vi "TCP.IP Client for Ripple Detection - Copy.vi"() -> ()   [LabVIEW 2021]
doc: "Demonstrates how to open a connection to an TCP server, read the data being sent, and display the data on a chart. This VI is designed to stop if the TCP connection is terminated."
panel:
  out "Filtered":dbl[](graph)
  out "Array Size 3":u32
  out "Delayed RMS2>RMS1 for 3 data":dynamicdata(graph)
  out "RMS2>RMS1 for 3 data":dynamicdata(graph)
  out "Array Size":u32
  out "RMS2>RMS1":dynamicdata(graph)
  out "RMS1":dynamicdata(graph)
  out "RMS2":dynamicdata(graph)
  out "Raw Data Collected":dynamicdata(graph)
  in  "Boolean":bool
  in  "Server Closed":string="The server VI closed the connection."
  out "Raw Data":dbl[](graph)
  in  "Stop":bool
  # "Overview: Demonstrates the use of the TCP functions to connect to a TCP server VI and receive data.\nInstructions:\n1. Ensure Simple TCP - Server.vi is already running.\n2. Run the VI.\n3. Click Stop to stop the VI. Note that if you stop the server VI, this VI will stop automatically."
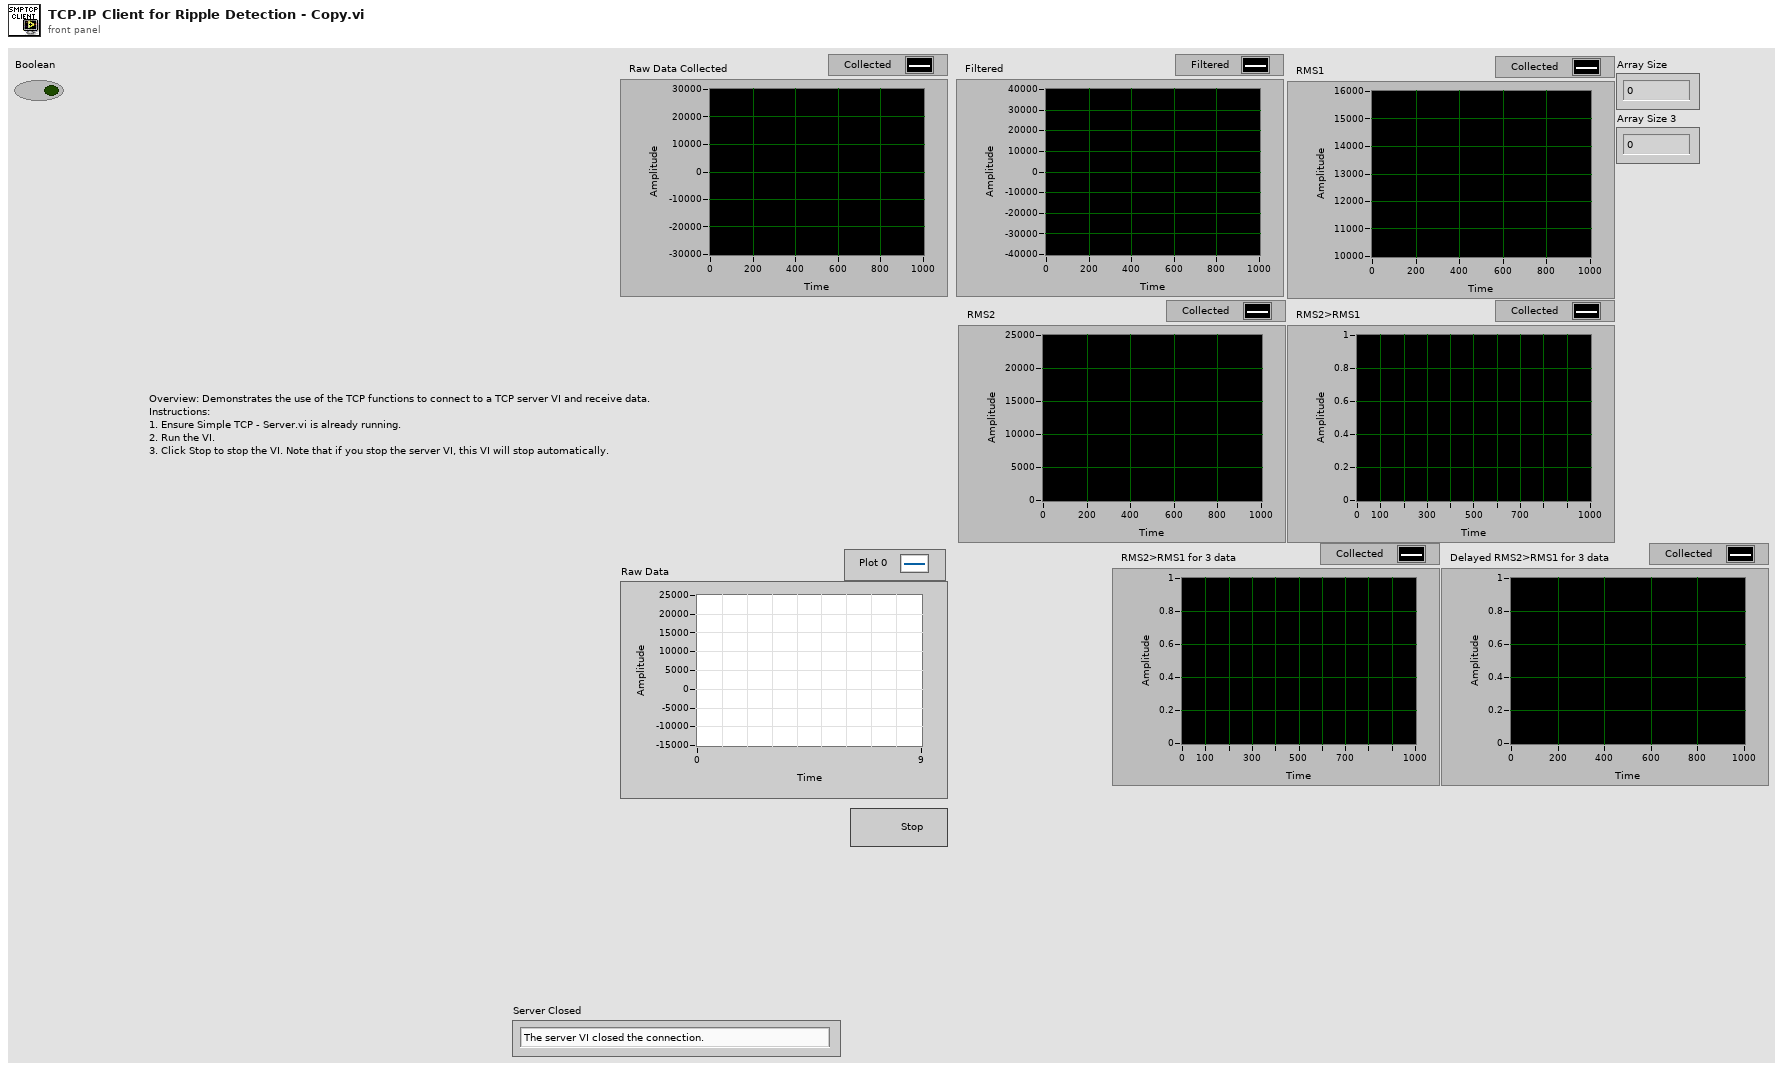
[diagram p1: front panel]
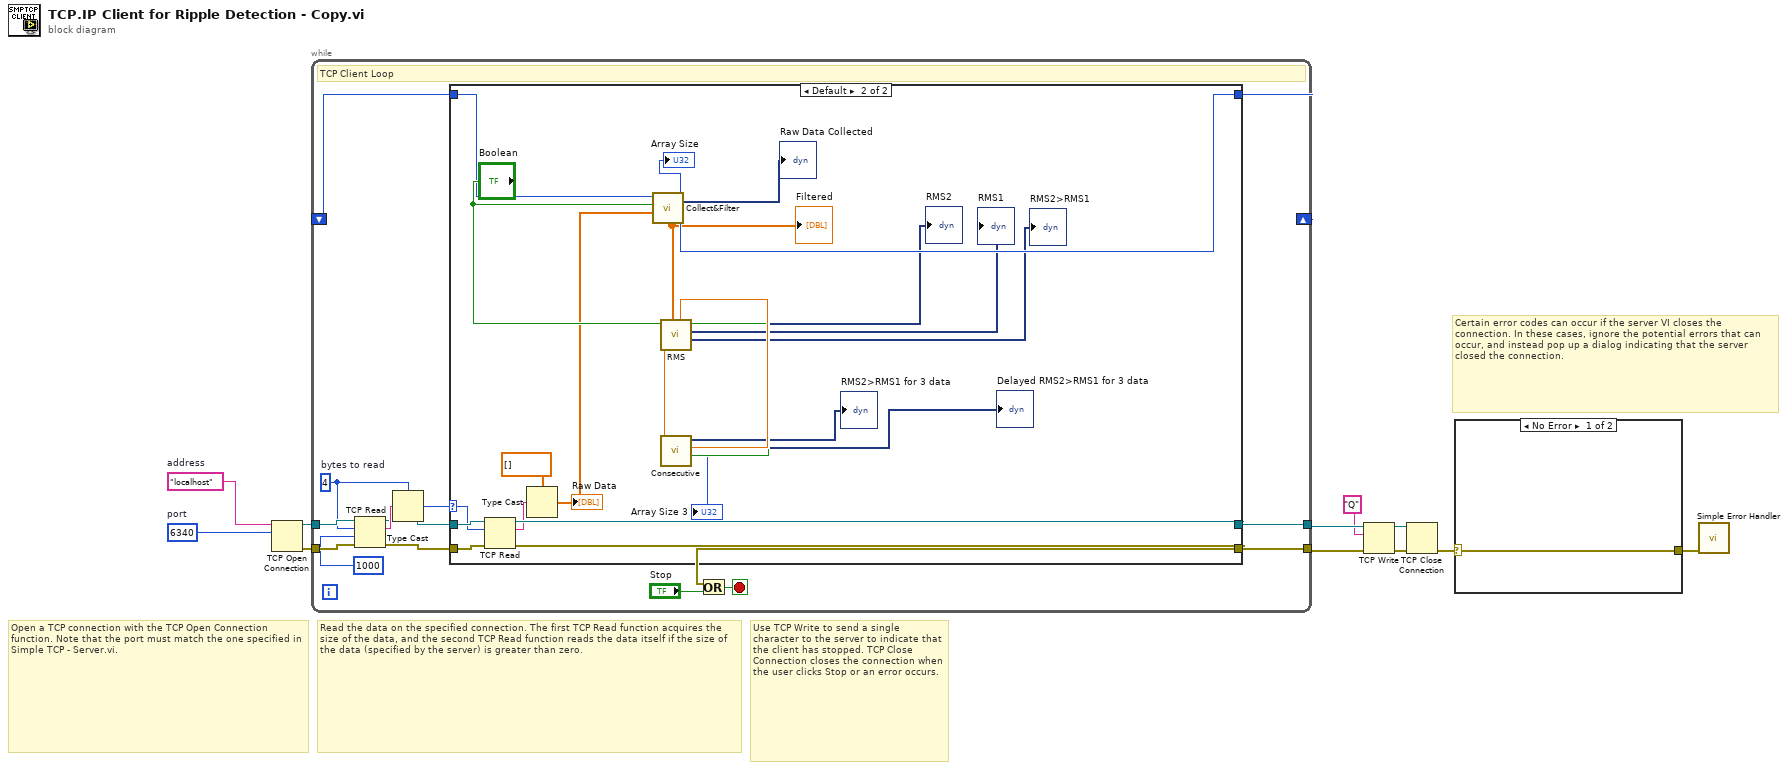
[diagram p0: block diagram]
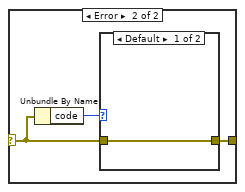
[diagram p2: hidden frame]
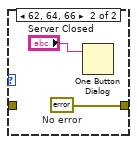
[diagram p3: hidden frame]
diagram:
  w1 = u16 6340  # port
  w2 = "localhost"  # address
  # "Certain error codes can occur if the server VI closes the connection. In these cases, ignore the potential errors that can occur, and instead pop up a dialog indicating that the server closed the connection."
  # "Use TCP Write to send a single character to the server to indicate that the client has stopped. TCP Close Connection closes the connection when the user clicks Stop or an error occurs."
  # "Read the data on the specified connection. The first TCP Read function acquires the size of the data, and the second TCP Read function reads the data itself if the size of the data (specified by the server) is greater than zero."
  # "Open a TCP connection with the TCP Open Connection function. Note that the port must match the one specified in Simple TCP - Server.vi."
  n1 = TCP Open Connection(address=w2, remote port or service name=w1) -> (connection ID=w11:refnum<k5>, error out=w10:errorcluster)  [unwired: 3 in]
  n2 = while {
    tunnel: w10 -> [w21]
    tunnel: w11 -> [w22]
    tunnel: [w17] -> w8
    tunnel: [w16] -> w6
    shift-right: [w12] -> _
    shift-left: _ -> [w13]
    stop <- w18 stop-if-true
    w20 = 4  # bytes to read
    # "TCP Client Loop"
    n3 = TCP Read(connection ID=w22, bytes to read=w20, error in (no error)=w21, 9:1000 ("timeout ms (25000)")) -> (connection ID out=w24:refnum<k5>, data out=w25:string, error out=w23:errorcluster)  [unwired: 1 in]
    n4 = Type Cast(type=w20, x=w25) -> (*(type *) &x=w15:i32)
    n5 = case shown="Default" w15 {
      selector: w15 -> [_ w44]
      tunnel: w24 -> [w28 w50]
      tunnel: w23 -> [w27 w49]
      tunnel: [w28 w47] -> w17
      tunnel: [w27 w46] -> w16
      tunnel: w13 -> [w26 w39]
      tunnel: [w26 w38] -> w12
      frame ..0 {
        # "The server has not written any data"
      }
      frame Default {
        n6 = TCP Read(connection ID=w50, bytes to read=w44, error in (no error)=w49) -> (connection ID out=w47:refnum<k5>, data out=w45:string, error out=w46:errorcluster)  [unwired: 2 in]
        n7 = Type Cast(type=dbl[] [] ("chart"), x=w45) -> (*(type *) &x=w37:dbl[])
        "Raw Data" <- w37
        n8 = call "Collect&Filter.vi"("chart"=w37, "Boolean"="Boolean", "Numeric in"=w39) -> ("Collected Signals"=→"Raw Data Collected":dynamicdata, "Numeric out"=w38:i32, "Array Size"=→"Array Size":u32, "Filtered X"=w29:dbl[])  [unwired: 5 in]
        "Filtered" <- w29
        n9 = call "RMS.vi"("Filtered X"=w29) -> ("RMS2>RMS1"=→"RMS2>RMS1":dynamicdata, "RMS1"=→"RMS1":dynamicdata, "RMS2"=→"RMS2":dynamicdata, "rms value 2"=w42:dbl, "rms value"=w41:dbl)  [unwired: 6 in]
        n10 = call "Consecutive.vi"("Boolean"="Boolean", "rms value"=w41, "rms value 2"=w42) -> ("Array Size 3"=→"Array Size 3":u32, "Delayed RMS2>RMS1 for 3 data"=→"Delayed RMS2>RMS1 for 3 data":dynamicdata, "RMS2>RMS1 for 3 data"=→"RMS2>RMS1 for 3 data":dynamicdata)  [unwired: 6 in]
      }
    }
    n11 = Or(x=w16, y="Stop") -> (x .or. y?=w18:bool)
  }
  n12 = TCP Write(connection ID=w8, data in="Q", error in (no error)=w6) -> (connection ID out=w9:refnum<k5>, error out=w7:errorcluster)  [unwired: 2 out]
  n13 = TCP Close Connection(connection ID=w9, error in (no error)=w7) -> (error out=w4:errorcluster)  [unwired: 1 in, 1 out]
  n14 = case shown="No Error" w4 {
    selector: w4 -> [w51 w53]
    tunnel: [w51 w52] -> w3
    frame No Error {
    }
    frame Error {
      n15 = Unbundle By Name(w53) -> ("code"=w54:i32)
      n16 = case shown="Default" w54 {
        tunnel: w53 -> [w55 _]
        tunnel: [w55 w57] -> w52
        frame Default {
        }
        frame 62, 64, 66 {
          w57 = errorcluster {"status"=FALSE, "code"=0, "source"=""}  # No error
          n17 = One Button Dialog(message="Server Closed") -> ()  [unwired: 1 in, 1 out]
        }
      }
    }
  }
  n18 = call <vilib>:"Simple Error Handler.vi"("error in (no error)"=w3) -> ()  [unwired: 4 in, 5 out]
